vi "runtest format timing.vi"(3 "POST (empty)":T1) -> (1 "$$TIMING$$":string)   [LabVIEW 2011]
uses:
  ITK EXT/utils/keyedarr.llb/Keyed Array.ctl
  ITK EXT/utils/strutil.llb/Case Matching.ctl
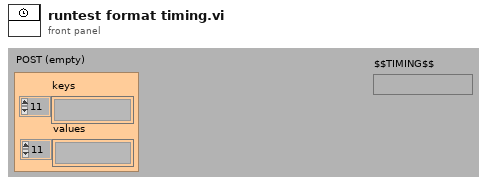
[diagram p1: front panel]
types:
  T1 = typedef "Keyed Array.ctl" = cluster{"keys":string[], "values":string[]}
  T2 = typedef "Case Matching.ctl" = enum16{"a != A", "a == A", "system"}
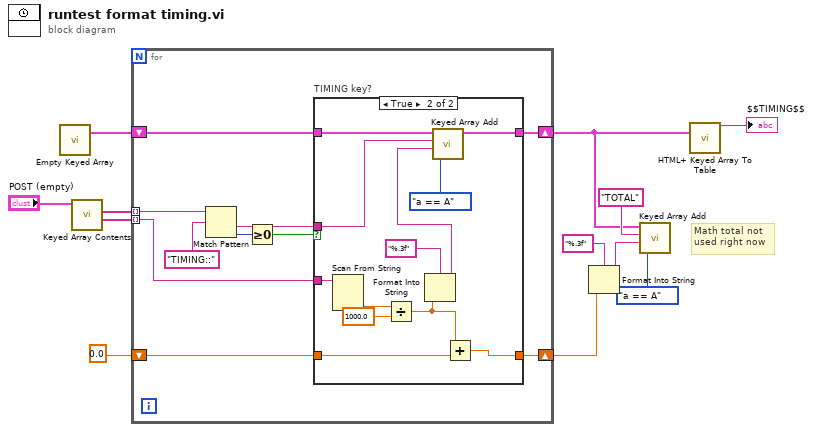
[diagram p0: block diagram]
diagram:
  # "Math total not\nused right now"
  n1 = call "Empty Keyed Array.vi"() -> ("empty keyed array"=w10:T1)  [unwired: 3 out]
  n2 = call "Keyed Array Contents.vi"("array in"="POST (empty)") -> ("values"=w8:string[], "keys"=w9:string[])  [unwired: 5 out]
  n3 = for {
    shift-right: [w17] -> w1
    shift-left: w10 -> [w18]
    tunnel: w9 -> [w22] mode=indexing
    tunnel: w8 -> [w15] mode=indexing
    shift-right: [w13] -> w3
    shift-left: 0.0 ("y") -> [w14]
    n4 = Match Pattern(string=w22, regular expression="TIMING::") -> (after substring=w16:string, offset past match=w20:i32)  [unwired: 3 out]
    n5 = Greater Or Equal To 0?(x=w20) -> (x >= 0?=w19:bool)
    n6 = case "TIMING key?" shown="True" w19 {
      tunnel: w18 -> [w24 w36]
      tunnel: [w24 w35] -> w17
      tunnel: w16 -> [_ w33]
      tunnel: w15 -> [_ w32]
      tunnel: w14 -> [w23 w26]
      tunnel: [w23 w25] -> w13
      frame False {
      }
      frame True {
        n7 = Scan From String(input string=w32) -> (output 1=w31:dbl)  [unwired: 3 in, 4 out]
        n8 = Divide(x=w31, y=1000.0) -> (x/y=w27:dbl)
        n9 = Format Into String(format string="%.3f", w27) -> (resulting string=w28:string)  [unwired: 2 in, 1 out]
        n10 = call "Keyed Array Add.vi"("case matching (sensitive)"=Case_Matching."a == A", "value"=w28, "key"=w33, "array in"=w36) -> ("array out"=w35:T1)  [unwired: 3 out]
        n11 = Add(x=w27, y=w26) -> (x+y=w25:dbl)
      }
    }
  }
  n12 = Format Into String(format string="%.3f", w3) -> (resulting string=w2:string)  [unwired: 2 in, 1 out]
  n13 = call "Keyed Array Add.vi"("case matching (sensitive)"=Case_Matching."a == A", "value"=w2, "key"="TOTAL", "array in"=w1) -> ()  [unwired: 4 out]
  n14 = call "HTML+ Keyed Array To Table.vi"("keyed array"=w1) -> ("HTML out"=→"$$TIMING$$":string)  [unwired: 3 in, 11 out]
